vi "Inteiros_OPC.vi"(11 "Numeric":i32) -> (0 "2-3":string, 3 "0-1":string)   [LabVIEW 2019]
panel:
  out "2-3":i32
  out "0-1":i32
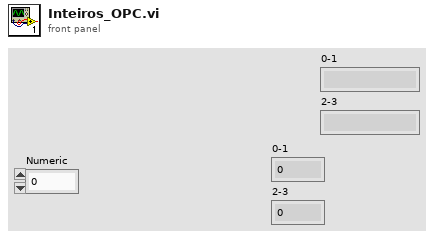
[diagram p1: front panel]
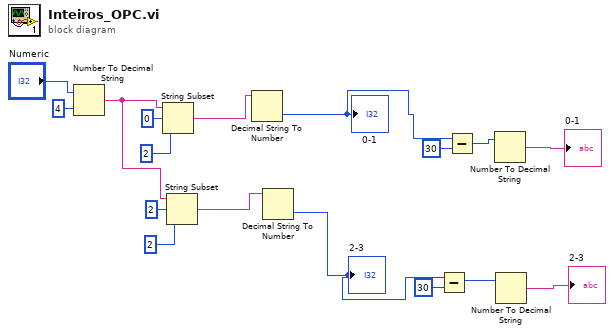
[diagram p0: block diagram]
diagram:
  n1 = Number To Decimal String(number="Numeric", width (-)=i16 4) -> (decimal integer string=w9:string)
  n2 = String Subset(string=w9, offset (0)=0, length (rest)=2 ("length (rest)")) -> (substring=w13:string)
  n3 = String Subset(string=w9, offset (0)=2, length (rest)=2 ("length (rest)")) -> (substring=w10:string)
  n4 = Decimal String To Number(string=w13) -> (number=w8:i32)  [unwired: 2 in, 1 out]
  "0-1" <- w8
  n5 = Decimal String To Number(string=w10) -> (number=w5:i32)  [unwired: 2 in, 1 out]
  "2-3" <- w5
  n6 = Subtract(x=w5, y=30) -> (x-y=w3:i32)
  n7 = Subtract(x=w8, y=30) -> (x-y=w4:i32)
  n8 = Number To Decimal String(number=w4) -> (decimal integer string=→"0-1":string)  [unwired: 1 in]
  n9 = Number To Decimal String(number=w3) -> (decimal integer string=→"2-3":string)  [unwired: 1 in]
